vi "Format&SaveDataCleanbckp.vi"(0 "Data_Angle_deg":sgl[](array[numeric])=[490.08, 490.12, 490.16, 490.2], 1 "Measurement type":T4(ring)=enum."Contrast", 2 "Spectrum Custom Mode":u16(ring)=1 caption="Detector" items=["PD 1", "APD 1", "APD 2", "APD 1+2", "PD 2"], 3 "Suppl_2D":dbl[][](array[numeric]), 4 "Params Save":T3, 5 "DotNum":dbl, 6 "Data_PLInt_cts":i32[](array[numeric])=[1, 3, 2, 1], 7 "Main 3D Data to write":dbl[][][](array[numeric])=[[[2.2, 4.4, 3.3, 5.5, 6.6]]], 10 "Params XY Map SubVI":T1, 11 "Suppl":dbl[](array[numeric]), 12 "Data_FSMPos_V":dbl[][](array[numeric]), 14 "Data_CCD_px":dbl[][](array[numeric]), 15 "L2Exc_deg":dbl[](array[numeric]), 17 "L2Det_deg":dbl[](array[numeric]), 19 "Suppl_3D":dbl[][][](array[numeric])) -> (9 "datasetnumber":string, 13 "Log File Out":string, 16 "FullComment":string, 18 "WrittenDatasetName":string)   [LabVIEW 2019]
uses:
  TypeDefs/AcqMode.ctl
  <vilib>/UPVI/lvhdf5/dataset.llb/LVH5D Operation.ctl
  <vilib>/Utility/miscctls.llb/LVRectTypeDef.ctl
  <vilib>/UPVI/lvhdf5/attribute.llb/LVH5A Operation.ctl
  <vilib>/UPVI/lvhdf5/group.llb/H5G_obj_t.ctl
  <vilib>/UPVI/lvhdf5/identifier.llb/Not an HDF5 Refnum Constant.vi
  <vilib>/UPVI/lvhdf5/common.llb/To HDF5 Ref.vi
  <vilib>/UPVI/lvhdf5/group.llb/OpenCreateGroup (String).vi
  <vilib>/Utility/VariantDataType/GetClusterInfo.vi
  <vilib>/Utility/VariantDataType/GetTypeInfo.vi
  <vilib>/UPVI/lvhdf5/utility.llb/Select HDF5 Dialog.vi
  <vilib>/UPVI/lvhdf5/utility.llb/Select HDF5 Dialog (Object Only).vi
  <vilib>/UPVI/lvhdf5/dataset.llb/Simple H5Dwrite (Variant).vi
  <vilib>/UPVI/lvhdf5/attribute.llb/Write Multiple Attributes.vi
  <vilib>/UPVI/lvhdf5/dataset.llb/H5Dclose.vi
  <vilib>/UPVI/lvhdf5/dataset.llb/Write Dataset with Attributes.xnode
  <vilib>/UPVI/lvhdf5/library.llb/HDF5 Ref.ctl
  <vilib>/UPVI/lvhdf5/attribute.llb/Cluster to Attribute Array.xnode
  <vilib>/Utility/error.llb/Error Cluster From Error Code.vi
  <vilib>/UPVI/lvhdf5/dataset.llb/OpenCreateReplace Dataset by Element Type.vi
  <vilib>/UPVI/lvhdf5/dataspace.llb/H5Sselect_hyperslab.vi
  <vilib>/UPVI/lvhdf5/dataset.llb/H5Dwrite (Variant).vi
  <vilib>/UPVI/lvhdf5/dataset.llb/H5Dget_space.vi
  <vilib>/UPVI/lvhdf5/attribute.llb/private/LVH5AwriteWDTAttrs.vi
  <vilib>/UPVI/lvhdf5/dataspace.llb/H5Sclose.vi
  <vilib>/UPVI/lvhdf5/file.llb/LVH5F Operation.ctl
  <vilib>/UPVI/lvhdf5/utility.llb/Select HDF5 Dialog (File and Object).vi
  <vilib>/Utility/VariantDataType/VariantType.lvlib
panel:
  out "resulting string":string
  out "XyMap Params 2":dbl[][](array[numeric])
  out "SamplePrep":string
  out "SynthSolv":string
  out "SynthPolymPerc":dbl
  out "SynthPolym":string
  out "SynthDilution":dbl
  out "SynthTemp":dbl
  out "SynthName":string
  out "SampleOf":string
  out "SamplePrepdate":timestamp
  out "Detector":string
  out "Marker":i8[](array[numeric])
  out "FSM":dbl[](array[numeric])
  out "Att":dbl[](array[numeric])
  out "AttY":dbl
  out "AttX":dbl
  out "AttZ":dbl
  out "MarkerY":i8
  out "MarkerX":i8
  out "FSMx":dbl
  out "FSMy":dbl
  out "Grating":string
  in  "ESource":enum16{"P", "CW", "SK"}(ring)
  in  "Acq Mode":T2=enum."Spectrum" caption="Acq mode"
  in  "Log File In":string
  out "File path":path=path "Cluster Attributes.hdf5"
  in  "DatasetName":string="test"
  in  "Main 2D Data to write":dbl[][](array[numeric])=[[2.2, 4.4, 3.3, 5.5, 6.6]]
  in  "Comment":string="This is a test"
  out "Date":string="2006-1-11"
  in  "T_K":dbl=5.0
  in  "EPow_uW":dbl=0.21
  in  "EWL_nm":dbl=450.0
  in  "Time_ms":dbl=500.0
  in  "Det_Mono1_EntSlit_mm":dbl=0.01
  in  "Det_Mono1_ExtSlit_mm":dbl=0.01
  in  "WL_nm":sgl[](array[numeric])=[490.08, 490.12, 490.16, 490.2]
  in  "MeasurementName":string
  in  "FileName":string="test"
  in  "Det_Mono1_CenterWL_nm":dbl=490.0
  out "Exists":bool
  out "Homonyms":string[](array[string])
  out "size(s)":i32
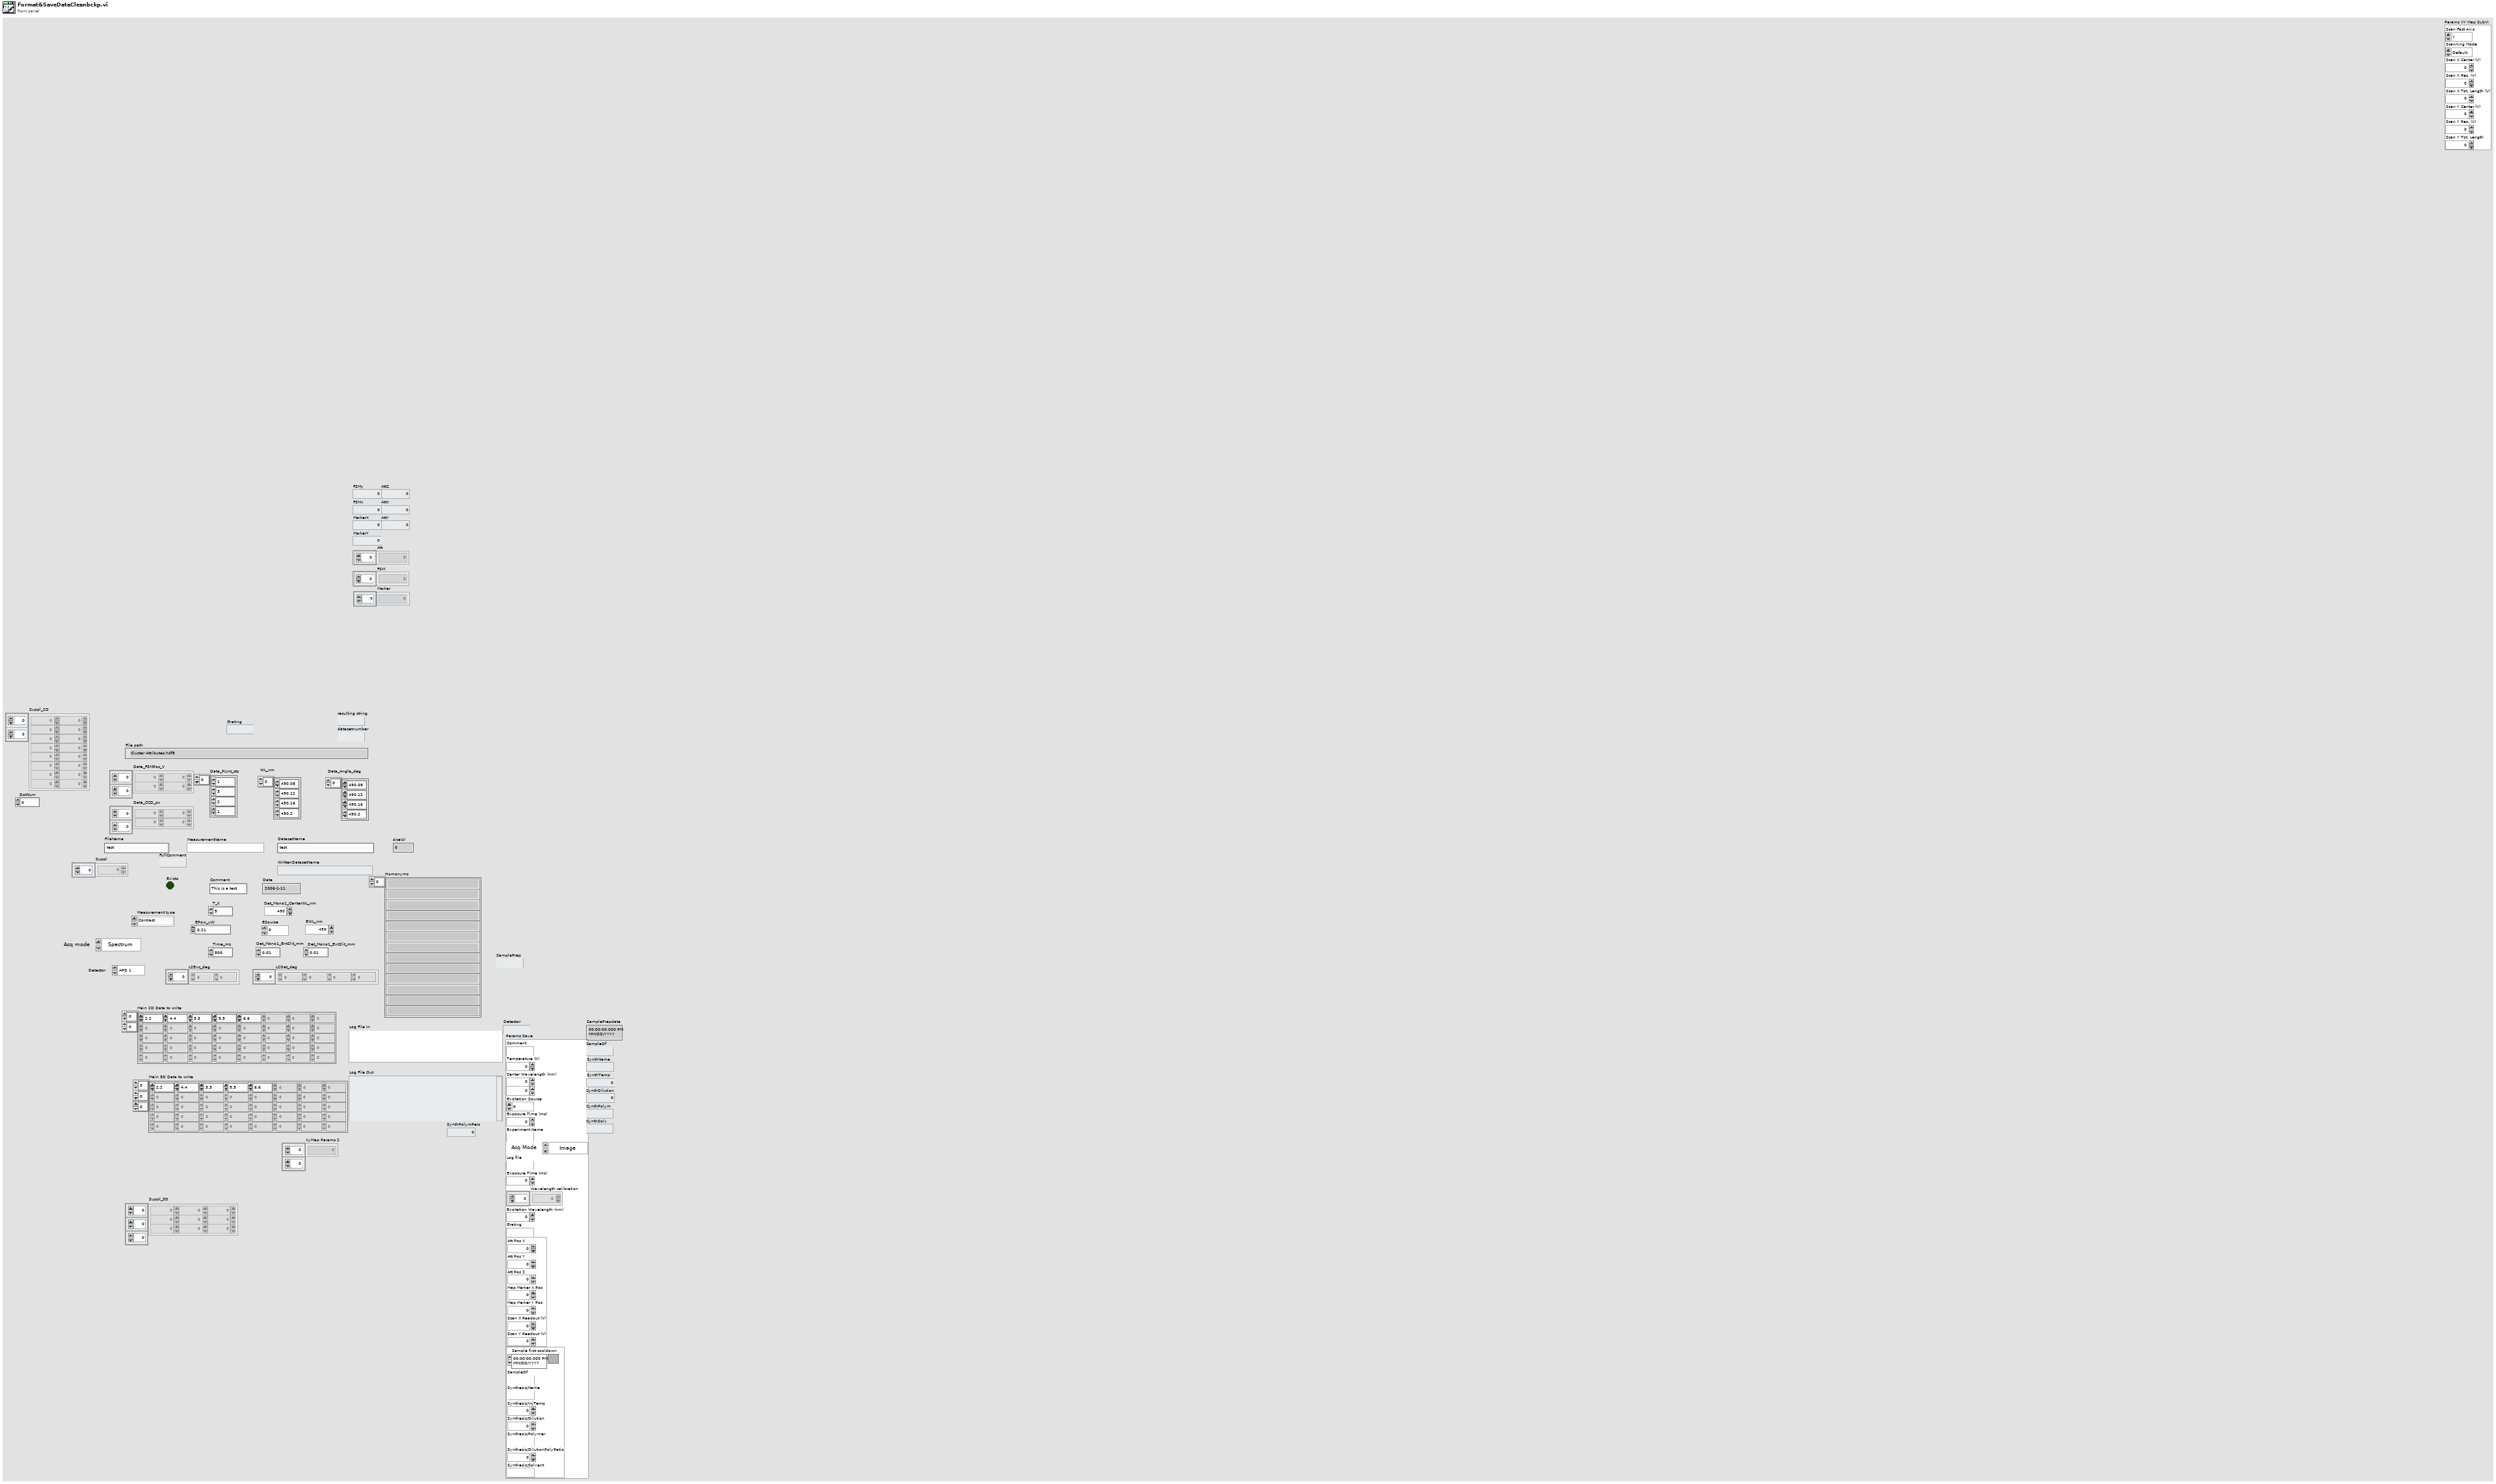
[diagram p1: front panel]
types:
  T1 = cluster{"Scan Fast Axis":enum16{"Y", "X"}, "Scanning Mode":enum16{"Default", "Snail", "Random", "Snake", "Line"}, "Scan X Center (V)":dbl, "Scan X Res. (V)":dbl, "Scan X Tot. Length (V)":dbl, "Scan Y Center (V)":dbl, "Scan Y Res. (V)":dbl, "Scan Y Tot. Length":dbl}
  T2 = typedef "AcqMode.ctl" = enum16{"Image", "Spectrum", "APD 1", "APD 2", "APD 1+2"}
  T3 = cluster{"Comment":string, "Temperature (K)":dbl, "Center Wavelength (nm)":dbl, "Numeric":dbl, "Excitation Source":enum16{"P", "CW", "SK"}, "Exposure Time (ms)":dbl, "Experiment Name":string, "Acq Mode":T2, "Log file":string, "Exposure Time (ms)":dbl, "Wavelength calibration":dbl[], "Excitation Wavelength (nm)":dbl, "Grating":string, "Cluster":cluster{"Att Pos X":dbl, "Att Pos Y":dbl, "Att Pos Z":dbl, "Map Marker X Pos":i8, "Map Marker Y Pos":i8, "Scan X Readout (V)":dbl, "Scan Y Readout (V)":dbl}, "Cluster":cluster{"Sample first cooldown":timestamp, "SampleOf":string, "Synthesis/Name":string, "Synthesis/InjTemp":dbl, "Synthesis/Dilution":dbl, "Synthesis/Polymer":string, "Synthesis/DilutionPolyRatio":dbl, "Synthesis/Solvent":string}}
  T4 = enum16{"Time Trace", "Contrast", "XY Intensity Map", "Polarisation", "Spectrum", "Michelson", "fPow", "PLE"}
  T5 = typedef "LVH5D Operation.ctl" = enum16{"open", "replace", "create", "open or create", "create or replace", "create or replace with confirmation"}
  T6 = typedef "LVH5A Operation.ctl" = enum16{"open", "replace", "create", "open or create", "create or replace", "create or replace with confirmation"}
  T7 = typedef "LVRectTypeDef.ctl" = cluster{"Left":i16, "Top":i16, "Right":i16, "Bottom":i16}
  T8 = cluster{"Behavior":enum32{"Invalid", "Default", "Floating", "Floating/Auto-Hide", "Modal"}, "Position":T7, "Center":bool, "Title":string}
  T9 = typedef "LVH5F Operation.ctl" = enum16{"open", "open or create", "create or replace", "create or replace (with confirmation)", "create", "open (read only)"}
  T10 = typedef "H5G_obj_t.ctl" = i32
  T11 = cluster{"Object Types (any)":T10[], "Object Pattern":string}
  T12 = cluster{"Att Pos X":dbl, "Att Pos Y":dbl, "Att Pos Z":dbl, "Map Marker X Pos":i8, "Map Marker Y Pos":i8, "Scan X Readout (V)":dbl, "Scan Y Readout (V)":dbl}
  T13 = cluster{"Sample first cooldown":timestamp, "SampleOf":string, "Synthesis/Name":string, "Synthesis/InjTemp":dbl, "Synthesis/Dilution":dbl, "Synthesis/Polymer":string, "Synthesis/DilutionPolyRatio":dbl, "Synthesis/Solvent":string}
  T14 = typedef "HDF5 Ref.ctl" = refnum<k1>
  T15 = cluster{"Date":string, "Comment":string, "T_K":dbl, "ESource":enum16{"P", "CW", "SK"}, "EWL_nm":dbl, "EPow_uW":dbl, "Time_ms":dbl, "WL_nm":sgl[], "Suppl":dbl[], "L2Exc_deg":dbl[], "L2Det_deg":dbl[], "Att":dbl[], "FSM":dbl[], "Marker":i8[], "Detector":string, "Grating":string, "SamplePrep":string, "SampleOf":string, "SynthName":string, "SynthTemp":dbl, "SynthDilution":dbl, "SynthPolym":string, "SynthPolymPerc":dbl, "SynthSolv":string}
  T16 = cluster{"Date":string, "Comment":string, "T_K":dbl, "ESource":enum16{"P", "CW", "SK"}, "EWL_nm":dbl, "EPow_uW":dbl, "Time_ms":dbl, "WL_nm":sgl[], "Suppl":dbl[], "L2Exc_deg":dbl[], "L2Det_deg":dbl[], "Suppl_2D":dbl[], "Att":dbl[], "FSM":dbl[], "Marker":i8[], "Detector":string, "Grating":string, "SamplePrep":string, "SampleOf":string, "SynthName":string, "SynthTemp":dbl, "SynthDilution":dbl, "SynthPolym":string, "SynthPolymPerc":dbl, "SynthSolv":string}
  T17 = cluster{"Date":string, "Comment":string, "T_K":dbl, "ESource":enum16{"P", "CW", "SK"}, "EWL_nm":dbl, "EPow_uW":dbl, "Time_ms":dbl, "WL_nm":sgl[], "Suppl":dbl[], "L2Exc_deg":dbl[], "L2Det_deg":dbl[], "Suppl_2D":dbl[][], "Att":dbl[], "FSM":dbl[], "Marker":i8[], "Detector":string, "Grating":string, "SamplePrep":string, "SampleOf":string, "SynthName":string, "SynthTemp":dbl, "SynthDilution":dbl, "SynthPolym":string, "SynthPolymPerc":dbl, "SynthSolv":string}
  T18 = cluster{"Date":string, "Comment":string, "T_K":dbl, "ESource":enum16{"P", "CW", "SK"}, "EWL_nm":dbl, "EPow_uW":dbl, "Time_ms":dbl, "WL_nm":sgl[], "Suppl_2D":dbl[][], "L2Exc_deg":dbl[], "L2Det_deg":dbl[], "Att":dbl[], "FSM":dbl[], "Marker":i8[], "Detector":string, "Grating":string, "SamplePrep":string, "SampleOf":string, "SynthName":string, "SynthTemp":dbl, "SynthDilution":dbl, "SynthPolym":string, "SynthPolymPerc":dbl, "SynthSolv":string}
  T19 = cluster{"Date":string, "Comment":string, "T_K":dbl, "ESource":enum16{"P", "CW", "SK"}, "EWL_nm":dbl, "EPow_uW":dbl, "Time_ms":dbl, "WL_nm":sgl[], "Suppl_3D":dbl[][][], "L2Exc_deg":dbl[], "L2Det_deg":dbl[], "Att":dbl[], "FSM":dbl[], "Marker":i8[], "Detector":string, "Grating":string, "SamplePrep":string, "SampleOf":string, "SynthName":string, "SynthTemp":dbl, "SynthDilution":dbl, "SynthPolym":string, "SynthPolymPerc":dbl, "SynthSolv":string}
  T20 = cluster{"Date":string, "Comment":string, "T_K":dbl, "ESource":enum16{"P", "CW", "SK"}, "EWL_nm":dbl, "EPow_uW":dbl, "Time_ms":dbl, "WL_nm":sgl[], "Suppl":dbl[], "L2Exc_deg":dbl[], "L2Det_deg":dbl[], "Att":dbl[], "FSM":dbl[], "Marker":i8[], "SamplePrep":string, "SampleOf":string, "SynthName":string, "SynthTemp":dbl, "SynthDilution":dbl, "SynthPolym":string, "SynthPolymPerc":dbl, "SynthSolv":string}
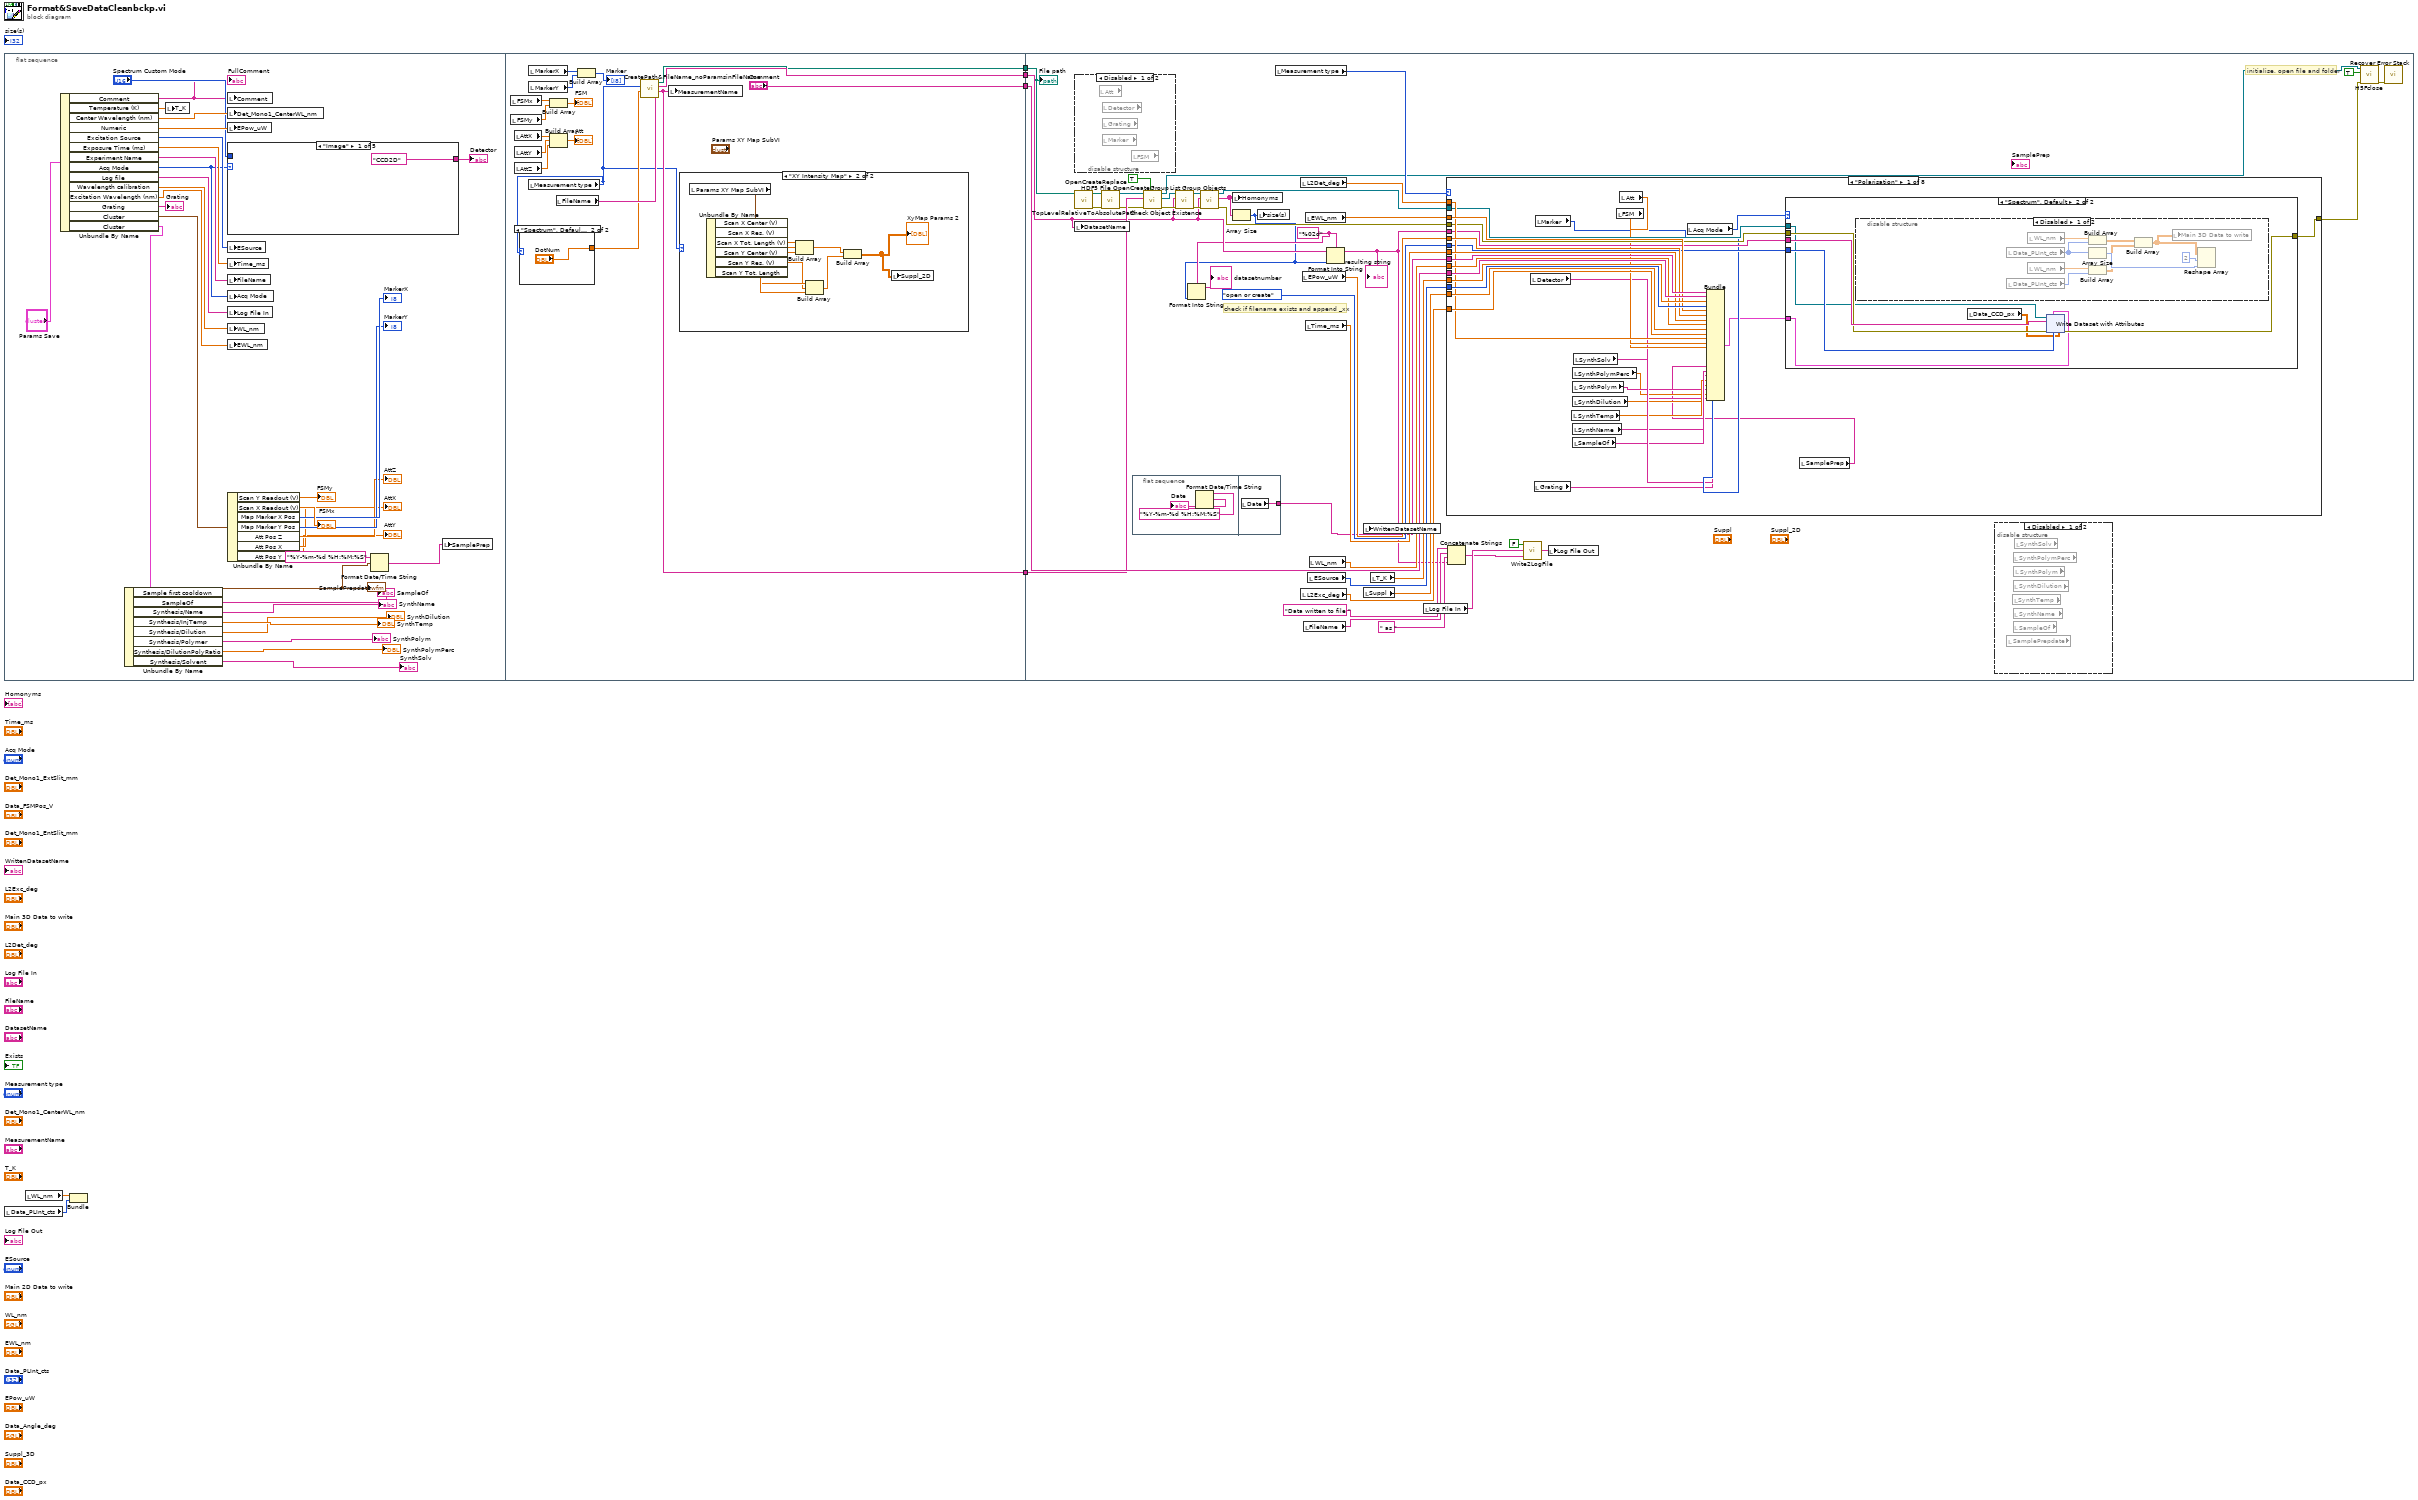
[diagram p0: block diagram]
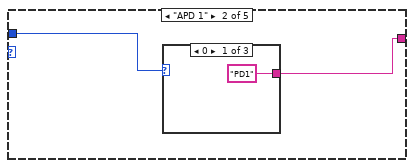
[diagram p2: hidden frame]
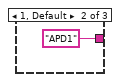
[diagram p3: hidden frame]
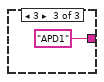
[diagram p4: hidden frame]
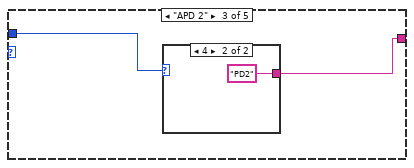
[diagram p5: hidden frame]
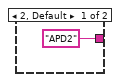
[diagram p6: hidden frame]
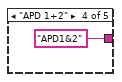
[diagram p7: hidden frame]
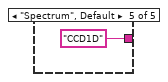
[diagram p8: hidden frame]
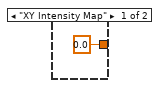
[diagram p9: hidden frame]
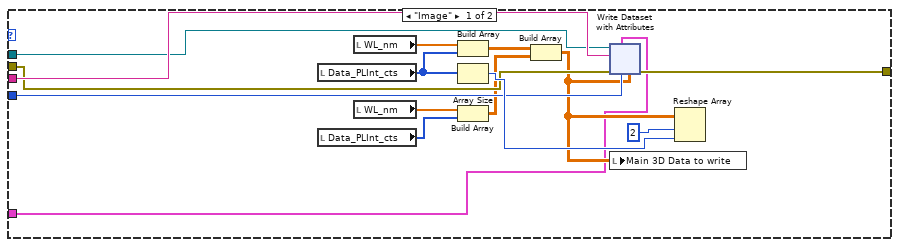
[diagram p13: hidden frame]
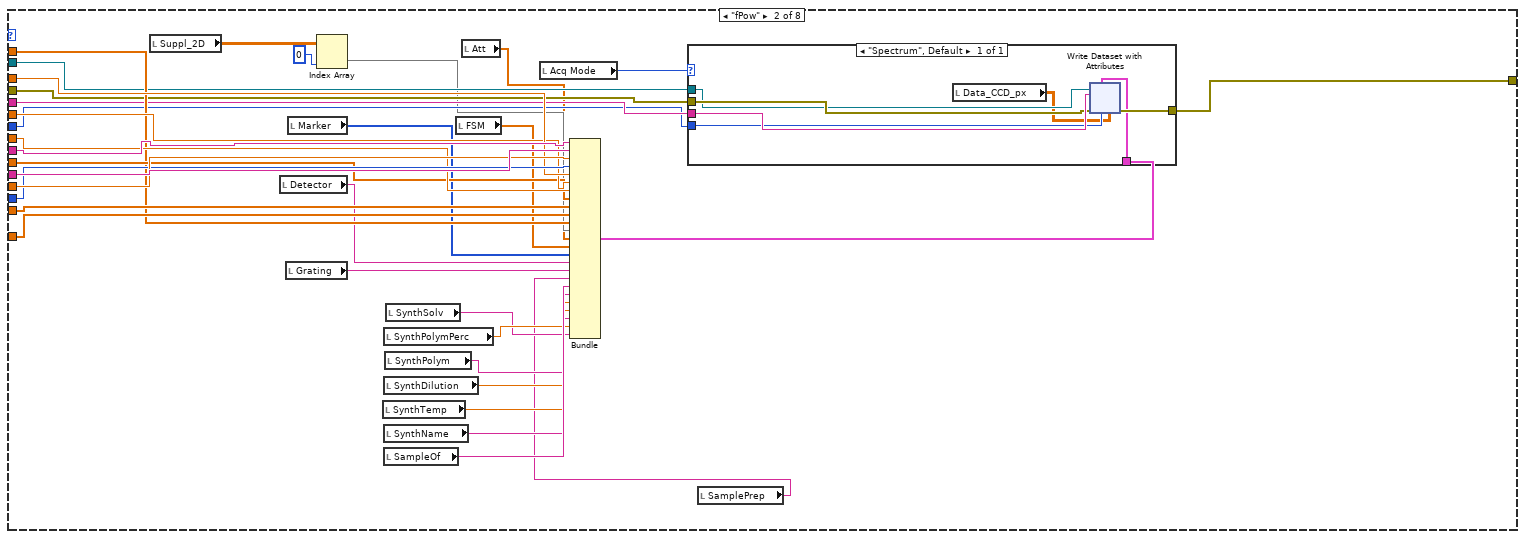
[diagram p15: hidden frame]
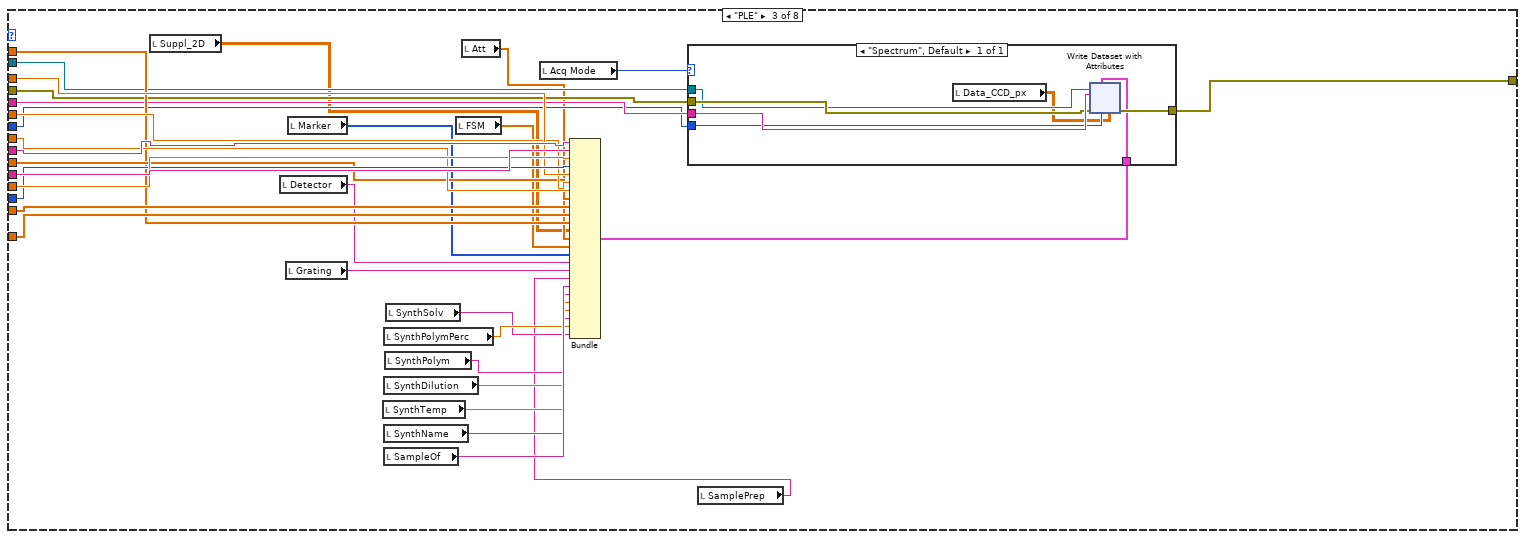
[diagram p16: hidden frame]
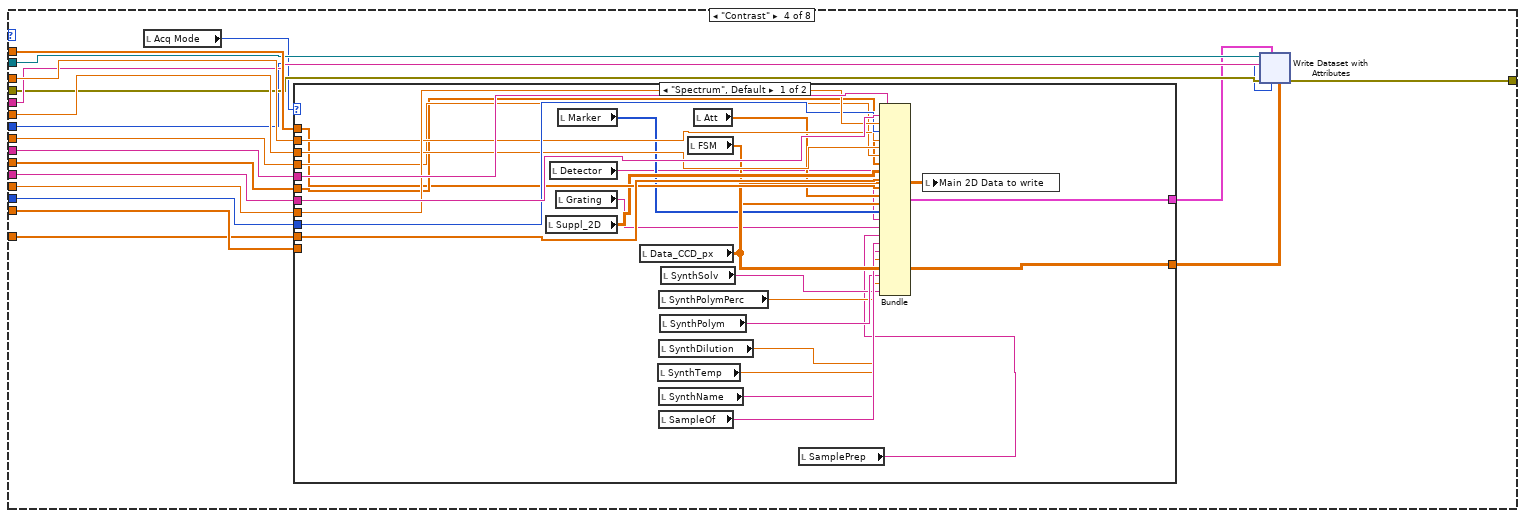
[diagram p17: hidden frame]
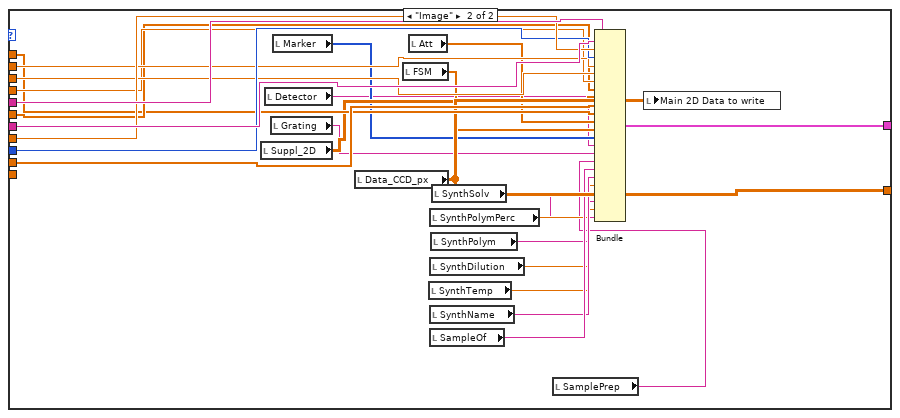
[diagram p18: hidden frame]
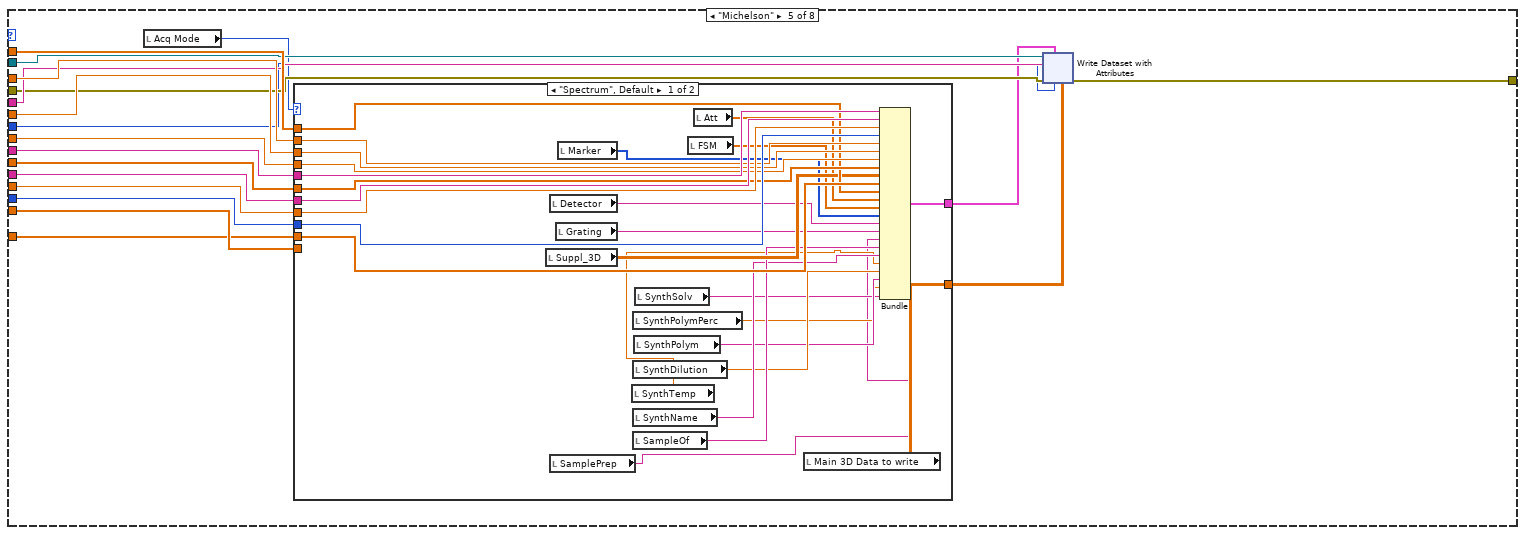
[diagram p19: hidden frame]
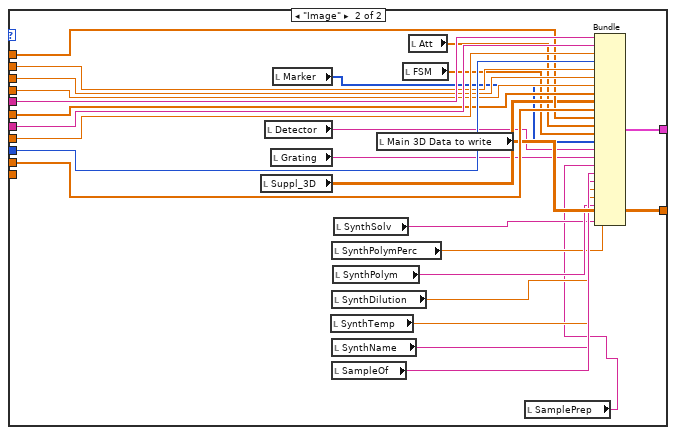
[diagram p20: hidden frame]
diagram:
  n1 = flat-sequence {
    tunnel: ["Comment"] -> w4
    tunnel: [w68] -> w3
    tunnel: [w67] -> w2
    tunnel: [w66] -> w1
    tunnel: w4 -> [w111]
    tunnel: w3 -> [w87]
    tunnel: w2 -> [w103]
    tunnel: w1 -> [w82]
    frame #0 {
      n2 = Unbundle By Name("Params Save") -> ("Comment"=w19:string, "Temperature (K)"=w40:dbl, "Center Wavelength (nm)"=w38:dbl, "Numeric"=w39:dbl, "Excitation Source"=w37:enum16{"P", "CW", "SK"}, "Exposure Time (ms)"=w36:dbl, "Experiment Name"=w34:string, "Acq Mode"=w31:T2, "Log file"=w35:string, "Wavelength calibration"=w32:dbl[], "Excitation Wavelength (nm)"=w33:dbl, "Grating"=→"Grating":string, "Cluster"=w27:T12, "Cluster"=w17:T13)
      "FullComment" <- w19
      n3 = Unbundle By Name(w17) -> ("Sample first cooldown"=w8:timestamp, "SampleOf"=→"SampleOf":string, "Synthesis/Name"=→"SynthName":string, "Synthesis/InjTemp"=→"SynthTemp":dbl, "Synthesis/Dilution"=→"SynthDilution":dbl, "Synthesis/Polymer"=→"SynthPolym":string, "Synthesis/DilutionPolyRatio"=→"SynthPolymPerc":dbl, "Synthesis/Solvent"=→"SynthSolv":string)
      "SamplePrepdate" <- w8
      n4 = local write "T_K"(w40) -> ()
      n5 = local write "Comment"(w19) -> ()
      n6 = local write "Det_Mono1_CenterWL_nm"(w38) -> ()
      n7 = local write "EPow_uW"(w39) -> ()
      n8 = case shown="\"Image\"" w31 {
        tunnel: ["CCD2D" w43 w48 "APD1&2" "CCD1D"] -> w29
        tunnel: "Spectrum Custom Mode" -> [_ w42 w47 _ _]
        frame "Image" {
        }
        frame "APD 1" {
          n9 = case shown="0" w42 {
            tunnel: ["PD1" "APD1" "APD1"] -> w43
            frame 0 {
            }
            frame 1, Default {
            }
            frame 3 {
            }
          }
        }
        frame "APD 2" {
          n10 = case shown="4" w47 {
            tunnel: ["APD2" "PD2"] -> w48
            frame 2, Default {
            }
            frame 4 {
            }
          }
        }
        frame "APD 1+2" {
        }
        frame "Spectrum", Default {
        }
      }
      "Detector" <- w29
      n11 = local write "ESource"(w37) -> ()
      n12 = local write "Time_ms"(w36) -> ()
      n13 = local write "FileName"(w34) -> ()
      n14 = local write "Acq Mode"(w31) -> ()
      n15 = local write "Log File In"(w35) -> ()
      n16 = local write "WL_nm"(w32) -> ()
      n17 = local write "EWL_nm"(w33) -> ()
      n18 = Unbundle By Name(w27) -> ("Scan Y Readout (V)"=→"FSMy":dbl, "Scan X Readout (V)"=→"FSMx":dbl, "Map Marker X Pos"=→"MarkerX":i8, "Map Marker Y Pos"=→"MarkerY":i8, "Att Pos Z"=→"AttZ":dbl, "Att Pos X"=→"AttX":dbl, "Att Pos Y"=→"AttY":dbl)
      n19 = Format Date/Time String(time format string (%c)="%Y-%m-%d %H:%M:%S", seconds (now)=w8) -> (date/time string=w7:string)  [unwired: 1 in]
      n20 = local write "SamplePrep"(w7) -> ()
    }
    frame #1 {
      n21 = local read "FSMx"() -> (w57:dbl)
      n22 = local read "FSMy"() -> (w58:dbl)
      n23 = local read "AttX"() -> (w54:dbl)
      n24 = local read "AttY"() -> (w55:dbl)
      n25 = local read "AttZ"() -> (w56:dbl)
      n26 = local read "Measurement type"() -> (w53:T4)
      n27 = case shown="\"Spectrum\", Default" w53 {
        tunnel: [0.0 ("DotNum") "DotNum"] -> w64
        frame "XY Intensity Map" {
        }
        frame "Spectrum", Default {
        }
      }
      n28 = local read "MarkerX"() -> (w59:i8)
      n29 = local read "MarkerY"() -> (w60:i8)
      n30 = Build Array(w57, w58) -> (→"FSM":dbl[])
      n31 = Build Array(w54, w55, w56) -> (→"Att":dbl[])
      n32 = local read "FileName"() -> (w65:string)
      n33 = Build Array(w59, w60) -> (→"Marker":i8[])
      n34 = call "CreatePath&FileName_noParamsinFileName.vi"("FileName"=w65, "DotNum"=w64, "Measurement type"=w53) -> ("MeasurementGroupName"=w67:string, "DatasetName"=w68:string, "File path"=w66:path)  [unwired: 3 in]
      n35 = local write "MeasurementName"(w67) -> ()
      n36 = case shown="\"XY Intensity Map\"" w53 {
        frame "Polarisation", Default {
        }
        frame "XY Intensity Map" {
          n37 = local read "Params XY Map SubVI"() -> (w81:T1)
          n38 = Unbundle By Name(w81) -> ("Scan X Center (V)"=w80:dbl, "Scan X Res. (V)"=w79:dbl, "Scan X Tot. Length (V)"=w78:dbl, "Scan Y Center (V)"=w76:dbl, "Scan Y Res. (V)"=w75:dbl, "Scan Y Tot. Length"=w77:dbl)
          n39 = Build Array(w80, w79, w78) -> (w74:dbl[])
          n40 = Build Array(w76, w75, w77) -> (w73:dbl[])
          n41 = Build Array(w74, w73) -> (w72:dbl[][])
          "XyMap Params 2" <- w72
          n42 = local write "Suppl_2D"(w72) -> ()
        }
      }
    }
    frame #2 {
      w85 = "%02d" ("format string")
      # "initialise, open file and folder"
      # "check if filename exists and append _xx"
      n43 = disable-structure shown="Disabled" {
        frame Disabled {
          n44 = local read "Att"() -> ()  [unwired: 1 out]
          n45 = local read "Detector"() -> ()  [unwired: 1 out]
          n46 = local read "Grating"() -> ()  [unwired: 1 out]
          n47 = local read "Marker"() -> ()  [unwired: 1 out]
          n48 = local read "FSM"() -> ()  [unwired: 1 out]
        }
        frame Enabled {
        }
      }
      n49 = call "TopLevelRelativeToAbsolutePath.vi"("Path Relative to Top Level VI"=w82) -> ("error out"=w96:errorcluster, "Absolute path"=w95:path)  [unwired: 9 in]
      n50 = local write "DatasetName"(w87) -> ()
      n51 = call <vilib>:"OpenCreateReplace HDF5 File.vi"("error in (no error)"=w96, "path"=w95) -> ("error out"=w98:errorcluster, "HDF5 Ref out"=w97:T14)  [unwired: 6 in]
      n52 = flat-sequence {
        tunnel: [w127] -> w110
        frame #0 {
          n53 = Format Date/Time String(time format string (%c)="%Y-%m-%d %H:%M:%S") -> (date/time string=→"Date":string)  [unwired: 2 in]
        }
        frame #1 {
          n54 = local read "Date"() -> (w127:string)
        }
      }
      n55 = call-poly <vilib>:"OpenCreateGroup.vi"("Create if not found (F)"=TRUE, "error in (no error)"=w98, "Group"=w103, "HDF5 Ref"=w97) -> ("error out"=w106:errorcluster, "HDF5 Group Ref"=w105:T14, "HDF5 Ref out"=w101:T14)  [unwired: 5 in]
      n56 = call <vilib>:"Check Object Existence.vi"("error in (no error)"=w106, "name"=w87, "HDF5 Ref"=w105) -> ("error out"=w107:errorcluster, "HDF5 Ref out"=w108:T14)  [unwired: 4 in, 1 out]
      n57 = call <vilib>:"List Group Objects.vi"("error in (no error)"=w107, "pattern"=w87, "HDF5 Loc Ref"=w108) -> ("error out"=w121:errorcluster, "Object Names"=w109:string[], "HDF5 Loc Ref out"=w123:T14)  [unwired: 3 in, 1 out]
      n58 = local write "Homonyms"(w109) -> ()
      n59 = Array Size(array=w109) -> (size(s)=w84:i32)
      n60 = Format Into String(format string=w85, w84) -> (resulting string=→"datasetnumber":string)  [unwired: 2 in, 1 out]
      n61 = local write "size(s)"(w84) -> ()
      n62 = local read "Measurement type"() -> (w102:T4)
      n63 = local read "L2Det_deg"() -> (w120:dbl[])
      n64 = local read "L2Exc_deg"() -> (w119:dbl[])
      n65 = local read "EPow_uW"() -> (w115:dbl)
      n66 = local read "FileName"() -> (w93:string)
      n67 = local read "EWL_nm"() -> (w114:dbl)
      n68 = local read "Time_ms"() -> (w116:dbl)
      n69 = local read "ESource"() -> (w113:enum16{"P", "CW", "SK"})
      n70 = local read "WL_nm"() -> (w117:sgl[])
      n71 = Format Into String(format string=w85, initial string=w87, w84) -> (resulting string=w91:string)  [unwired: 1 in, 1 out]
      "resulting string" <- w91
      n72 = local write "WrittenDatasetName"(w91) -> ()
      n73 = local read "Suppl"() -> (w118:dbl[])
      n74 = local read "T_K"() -> (w112:dbl)
      n75 = local read "Log File In"() -> (w90:string)
      n76 = case shown="\"Polarisation\"" w102 {
        tunnel: w110 -> [w158 w903 w1284 w1652 w2063 w2472 w4298 w5066]
        tunnel: w111 -> [w157 w902 w1283 w1651 w2062 w2471 w4297 w5065]
        tunnel: w112 -> [w156 w901 w1282 w1650 w2061 w2470 w4296 w5064]
        tunnel: w113 -> [w155 w900 w1281 w1649 w2060 w2469 w4295 w5063]
        tunnel: w114 -> [w154 w899 w1280 w1648 w2059 w2468 w4294 w5062]
        tunnel: w115 -> [w153 w898 w1279 w1647 w2058 w2467 w4293 w5061]
        tunnel: w116 -> [w152 w897 w1278 w1646 w2057 w2466 w4292 w5060]
        tunnel: w117 -> [w151 w896 w1277 w1645 w2056 w2465 w4291 w5059]
        tunnel: w118 -> [w150 w895 w1276 w1644 w2055 w2464 w4290 w5058]
        tunnel: w119 -> [w149 w894 w1275 w1643 w2054 w2463 w4289 w5057]
        tunnel: w120 -> [w148 w893 w1274 w1642 w2053 w2462 w4288 w5056]
        tunnel: w91 -> [w147 w892 w1273 w1641 w2052 w2461 w4287 w5055]
        tunnel: w121 -> [w146 w891 w1272 w1640 w2051 w2460 w4286 w5054]
        tunnel: LVH5D_Operation."open or create" ("operation (open or create)") -> [w145 w890 w1271 w1639 w2050 w2459 w4285 w5053]
        tunnel: w123 -> [w144 w889 w1270 w1638 w2049 w2458 w4284 w5052]
        tunnel: [w143 w888 w1269 w1637 w2048 w2457 w4283 w5051] -> w124
        frame "Polarisation" {
          n77 = local read "Detector"() -> (w138:string)
          n78 = local read "Grating"() -> (w137:string)
          n79 = local read "Marker"() -> (w139:i8[])
          n80 = local read "SynthTemp"() -> (w134:dbl)
          n81 = local read "SynthPolymPerc"() -> (w131:dbl)
          n82 = local read "SynthDilution"() -> (w133:dbl)
          n83 = local read "SynthName"() -> (w135:string)
          n84 = local read "SampleOf"() -> (w136:string)
          n85 = local read "SynthPolym"() -> (w132:string)
          n86 = local read "SynthSolv"() -> (w130:string)
          n87 = local read "FSM"() -> (w140:dbl[])
          n88 = local read "Att"() -> (w141:dbl[])
          n89 = local read "Acq Mode"() -> (w142:T2)
          n90 = local read "SamplePrep"() -> (w128:string)
          n91 = Bundle("Date"=w158, "Comment"=w157, "T_K"=w156, "ESource"=w155, "EWL_nm"=w154, "EPow_uW"=w153, "Time_ms"=w152, "WL_nm"=w151, "Suppl"=w150, "L2Exc_deg"=w149, "L2Det_deg"=w148, "Att"=w141, "FSM"=w140, "Marker"=w139, "Detector"=w138, "Grating"=w137, "SamplePrep"=w128, "SampleOf"=w136, "SynthName"=w135, "SynthTemp"=w134, "SynthDilution"=w133, "SynthPolym"=w132, "SynthPolymPerc"=w131, "SynthSolv"=w130) -> (w129:T15)  [unwired: 1 in]
          n92 = case shown="\"Spectrum\", Default" w142 {
            tunnel: w147 -> [w169 w520]
            tunnel: w146 -> [w168 w519]
            tunnel: w145 -> [w167 w518]
            tunnel: w144 -> [w166 w517]
            tunnel: [w165 w516] -> w143
            tunnel: w129 -> [w159 w514]
            frame "Image" {
              n93 = local read "Data_PLInt_cts"() -> (w171:i32[])
              n94 = local read "Data_PLInt_cts"() -> (w163:i32[])
              n95 = local read "WL_nm"() -> (w170:sgl[])
              n96 = local read "WL_nm"() -> (w164:sgl[])
              n97 = Build Array(w170, w171) -> (w161:sgl[][])
              n98 = Array Size(array=w171) -> (size(s)=w172:i32)
              n99 = Build Array(w164, w163) -> (w162:sgl[][])
              n100 = Build Array(w161, w162) -> (w160:sgl[][][])
              n101 = xnode "Write Dataset with Attributes"("Dataset Path"=w169, "error in (no error)"=w168, "operation (open or create)"=w167, "HDF5 Path or Ref"=w166, "Attribute Value(s)"=w159, "Data"=w160) -> ("error out"=w165:errorcluster)  [unwired: 2 in, 2 out]
              n102 = local write "Main 3D Data to write"(w160) -> ()
              n103 = Reshape Array(w160, 2 ("dimension size"), w172) -> ()  [unwired: 1 out]
            }
            frame "Spectrum", Default {
              n104 = disable-structure shown="Disabled" {
                frame Disabled {
                  n105 = local read "Data_PLInt_cts"() -> (w527:i32[])
                  n106 = local read "Data_PLInt_cts"() -> (w524:i32[])
                  n107 = local read "WL_nm"() -> (w526:sgl[])
                  n108 = local read "WL_nm"() -> (w525:sgl[])
                  n109 = Build Array(w526, w527) -> (w522:sgl[][])
                  n110 = Array Size(array=w527) -> (size(s)=w528:i32)
                  n111 = Build Array(w525, w524) -> (w523:sgl[][])
                  n112 = Build Array(w522, w523) -> (w521:sgl[][][])
                  n113 = local write "Main 3D Data to write"(w521) -> ()
                  n114 = Reshape Array(w521, 2 ("dimension size"), w528) -> ()  [unwired: 1 out]
                }
                frame Enabled {
                }
              }
              n115 = local read "Data_CCD_px"() -> (w515:dbl[][])
              n116 = xnode "Write Dataset with Attributes"("Dataset Path"=w520, "error in (no error)"=w519, "operation (open or create)"=w518, "HDF5 Path or Ref"=w517, "Attribute Value(s)"=w514, "Data"=w515) -> ("error out"=w516:errorcluster)  [unwired: 2 in, 2 out]
            }
          }
        }
        frame "fPow" {
          n117 = local read "Suppl_2D"() -> (w886:dbl[][])
          n118 = local read "Detector"() -> (w880:string)
          n119 = local read "Grating"() -> (w879:string)
          n120 = local read "Marker"() -> (w881:i8[])
          n121 = Index Array(array=w886, index (col)=0 ("disabled index (col)")) -> (element=w884:dbl[])  [unwired: 1 in]
          n122 = local read "SynthTemp"() -> (w876:dbl)
          n123 = local read "SynthPolymPerc"() -> (w873:dbl)
          n124 = local read "SynthDilution"() -> (w875:dbl)
          n125 = local read "SynthName"() -> (w877:string)
          n126 = local read "SampleOf"() -> (w878:string)
          n127 = local read "SynthPolym"() -> (w874:string)
          n128 = local read "SynthSolv"() -> (w872:string)
          n129 = local read "FSM"() -> (w882:dbl[])
          n130 = local read "Att"() -> (w883:dbl[])
          n131 = local read "Acq Mode"() -> (w887:T2)
          n132 = local read "SamplePrep"() -> (w870:string)
          n133 = Bundle("Date"=w903, "Comment"=w902, "T_K"=w901, "ESource"=w900, "EWL_nm"=w899, "EPow_uW"=w898, "Time_ms"=w897, "WL_nm"=w896, "Suppl"=w895, "L2Exc_deg"=w894, "L2Det_deg"=w893, "Suppl_2D"=w884, "Att"=w883, "FSM"=w882, "Marker"=w881, "Detector"=w880, "Grating"=w879, "SamplePrep"=w870, "SampleOf"=w878, "SynthName"=w877, "SynthTemp"=w876, "SynthDilution"=w875, "SynthPolym"=w874, "SynthPolymPerc"=w873, "SynthSolv"=w872) -> (w871:T16)  [unwired: 1 in]
          n134 = case shown="\"Spectrum\", Default" w887 {
            tunnel: w892 -> [w910]
            tunnel: w891 -> [w909]
            tunnel: w890 -> [w908]
            tunnel: w889 -> [w907]
            tunnel: [w906] -> w888
            tunnel: w871 -> [w904]
            frame "Spectrum", Default {
              n135 = local read "Data_CCD_px"() -> (w905:dbl[][])
              n136 = xnode "Write Dataset with Attributes"("Dataset Path"=w910, "error in (no error)"=w909, "operation (open or create)"=w908, "HDF5 Path or Ref"=w907, "Attribute Value(s)"=w904, "Data"=w905) -> ("error out"=w906:errorcluster)  [unwired: 2 in, 2 out]
            }
          }
        }
        frame "PLE" {
          n137 = local read "Suppl_2D"() -> (w1254:dbl[][])
          n138 = local read "Detector"() -> (w1264:string)
          n139 = local read "Grating"() -> (w1263:string)
          n140 = local read "Marker"() -> (w1265:i8[])
          n141 = local read "SynthTemp"() -> (w1260:dbl)
          n142 = local read "SynthPolymPerc"() -> (w1257:dbl)
          n143 = local read "SynthDilution"() -> (w1259:dbl)
          n144 = local read "SynthName"() -> (w1261:string)
          n145 = local read "SampleOf"() -> (w1262:string)
          n146 = local read "SynthPolym"() -> (w1258:string)
          n147 = local read "SynthSolv"() -> (w1256:string)
          n148 = local read "FSM"() -> (w1266:dbl[])
          n149 = local read "Att"() -> (w1267:dbl[])
          n150 = local read "Acq Mode"() -> (w1268:T2)
          n151 = local read "SamplePrep"() -> (w1255:string)
          n152 = Bundle("Date"=w1284, "Comment"=w1283, "T_K"=w1282, "ESource"=w1281, "EWL_nm"=w1280, "EPow_uW"=w1279, "Time_ms"=w1278, "WL_nm"=w1277, "Suppl"=w1276, "L2Exc_deg"=w1275, "L2Det_deg"=w1274, "Suppl_2D"=w1254, "Att"=w1267, "FSM"=w1266, "Marker"=w1265, "Detector"=w1264, "Grating"=w1263, "SamplePrep"=w1255, "SampleOf"=w1262, "SynthName"=w1261, "SynthTemp"=w1260, "SynthDilution"=w1259, "SynthPolym"=w1258, "SynthPolymPerc"=w1257, "SynthSolv"=w1256) -> (w1253:T17)  [unwired: 1 in]
          n153 = case shown="\"Spectrum\", Default" w1268 {
            tunnel: w1273 -> [w1291]
            tunnel: w1272 -> [w1290]
            tunnel: w1271 -> [w1289]
            tunnel: w1270 -> [w1288]
            tunnel: [w1287] -> w1269
            tunnel: w1253 -> [w1285]
            frame "Spectrum", Default {
              n154 = local read "Data_CCD_px"() -> (w1286:dbl[][])
              n155 = xnode "Write Dataset with Attributes"("Dataset Path"=w1291, "error in (no error)"=w1290, "operation (open or create)"=w1289, "HDF5 Path or Ref"=w1288, "Attribute Value(s)"=w1285, "Data"=w1286) -> ("error out"=w1287:errorcluster)  [unwired: 2 in, 2 out]
            }
          }
        }
        frame "Contrast" {
          n156 = local read "Acq Mode"() -> (w1635:T2)
          n157 = case shown="\"Spectrum\", Default" w1635 {
            tunnel: w1652 -> [w1678 w1704]
            tunnel: w1651 -> [w1677 w1703]
            tunnel: w1650 -> [w1676 w1702]
            tunnel: w1649 -> [w1675 w1701]
            tunnel: w1648 -> [w1674 w1700]
            tunnel: w1647 -> [w1673 w1699]
            tunnel: w1646 -> [w1672 w1698]
            tunnel: w1645 -> [w1671 w1697]
            tunnel: w1644 -> [_ _]
            tunnel: w1643 -> [w1670 w1696]
            tunnel: w1642 -> [w1669 w1695]
            tunnel: [w1668 w1694] -> w1636
            tunnel: [w1654 w1680] -> w1634
            frame "Spectrum", Default {
              n158 = local read "Suppl_2D"() -> (w1667:dbl[][])
              n159 = local read "Detector"() -> (w1663:string)
              n160 = local read "Grating"() -> (w1662:string)
              n161 = local read "Marker"() -> (w1664:i8[])
              n162 = local read "Data_CCD_px"() -> (w1668:dbl[][])
              n163 = local read "SynthTemp"() -> (w1659:dbl)
              n164 = local read "SynthPolymPerc"() -> (w1656:dbl)
              n165 = local read "SynthDilution"() -> (w1658:dbl)
              n166 = local read "SynthName"() -> (w1660:string)
              n167 = local read "SampleOf"() -> (w1661:string)
              n168 = local read "SynthPolym"() -> (w1657:string)
              n169 = local read "SynthSolv"() -> (w1655:string)
              n170 = local read "FSM"() -> (w1665:dbl[])
              n171 = local read "Att"() -> (w1666:dbl[])
              n172 = local read "SamplePrep"() -> (w1653:string)
              n173 = Bundle("Date"=w1678, "Comment"=w1677, "T_K"=w1676, "ESource"=w1675, "EWL_nm"=w1674, "EPow_uW"=w1673, "Time_ms"=w1672, "WL_nm"=w1671, "Suppl_2D"=w1667, "L2Exc_deg"=w1670, "L2Det_deg"=w1669, "Att"=w1666, "FSM"=w1665, "Marker"=w1664, "Detector"=w1663, "Grating"=w1662, "SamplePrep"=w1653, "SampleOf"=w1661, "SynthName"=w1660, "SynthTemp"=w1659, "SynthDilution"=w1658, "SynthPolym"=w1657, "SynthPolymPerc"=w1656, "SynthSolv"=w1655) -> (w1654:T18)  [unwired: 1 in]
              n174 = local write "Main 2D Data to write"(w1668) -> ()
            }
            frame "Image" {
              n175 = local read "Suppl_2D"() -> (w1693:dbl[][])
              n176 = local read "Detector"() -> (w1689:string)
              n177 = local read "Grating"() -> (w1688:string)
              n178 = local read "Marker"() -> (w1690:i8[])
              n179 = local read "Data_CCD_px"() -> (w1694:dbl[][])
              n180 = local read "FSM"() -> (w1691:dbl[])
              n181 = local read "Att"() -> (w1692:dbl[])
              n182 = local read "SynthTemp"() -> (w1685:dbl)
              n183 = local read "SynthPolymPerc"() -> (w1682:dbl)
              n184 = local read "SynthDilution"() -> (w1684:dbl)
              n185 = local read "SynthName"() -> (w1686:string)
              n186 = local read "SampleOf"() -> (w1687:string)
              n187 = local read "SynthPolym"() -> (w1683:string)
              n188 = local read "SynthSolv"() -> (w1681:string)
              n189 = local read "SamplePrep"() -> (w1679:string)
              n190 = Bundle("Date"=w1704, "Comment"=w1703, "T_K"=w1702, "ESource"=w1701, "EWL_nm"=w1700, "EPow_uW"=w1699, "Time_ms"=w1698, "WL_nm"=w1697, "Suppl_2D"=w1693, "L2Exc_deg"=w1696, "L2Det_deg"=w1695, "Att"=w1692, "FSM"=w1691, "Marker"=w1690, "Detector"=w1689, "Grating"=w1688, "SamplePrep"=w1679, "SampleOf"=w1687, "SynthName"=w1686, "SynthTemp"=w1685, "SynthDilution"=w1684, "SynthPolym"=w1683, "SynthPolymPerc"=w1682, "SynthSolv"=w1681) -> (w1680:T18)  [unwired: 1 in]
              n191 = local write "Main 2D Data to write"(w1694) -> ()
            }
          }
          n192 = xnode "Write Dataset with Attributes"("Dataset Path"=w1641, "error in (no error)"=w1640, "operation (open or create)"=w1639, "HDF5 Path or Ref"=w1638, "Attribute Value(s)"=w1634, "Data"=w1636) -> ("error out"=w1637:errorcluster)  [unwired: 2 in, 2 out]
        }
        frame "Michelson" {
          n193 = local read "Acq Mode"() -> (w2046:T2)
          n194 = case shown="\"Spectrum\", Default" w2046 {
            tunnel: w2063 -> [w2089 w2115]
            tunnel: w2062 -> [w2088 w2114]
            tunnel: w2061 -> [w2087 w2113]
            tunnel: w2060 -> [w2086 w2112]
            tunnel: w2059 -> [w2085 w2111]
            tunnel: w2058 -> [w2084 w2110]
            tunnel: w2057 -> [w2083 w2109]
            tunnel: w2056 -> [w2082 w2108]
            tunnel: w2055 -> [_ _]
            tunnel: w2054 -> [w2081 w2107]
            tunnel: w2053 -> [w2080 w2106]
            tunnel: [w2079 w2105] -> w2047
            tunnel: [w2065 w2091] -> w2045
            frame "Spectrum", Default {
              n195 = local read "Suppl_3D"() -> (w2078:dbl[][][])
              n196 = local read "Detector"() -> (w2074:string)
              n197 = local read "SamplePrep"() -> (w2064:string)
              n198 = local read "Grating"() -> (w2073:string)
              n199 = local read "Marker"() -> (w2075:i8[])
              n200 = local read "SynthTemp"() -> (w2070:dbl)
              n201 = local read "SynthPolymPerc"() -> (w2067:dbl)
              n202 = local read "SynthDilution"() -> (w2069:dbl)
              n203 = local read "SynthName"() -> (w2071:string)
              n204 = local read "SampleOf"() -> (w2072:string)
              n205 = local read "SynthPolym"() -> (w2068:string)
              n206 = local read "SynthSolv"() -> (w2066:string)
              n207 = local read "FSM"() -> (w2076:dbl[])
              n208 = local read "Att"() -> (w2077:dbl[])
              n209 = local read "Main 3D Data to write"() -> (w2079:dbl[][][])
              n210 = Bundle("Date"=w2089, "Comment"=w2088, "T_K"=w2087, "ESource"=w2086, "EWL_nm"=w2085, "EPow_uW"=w2084, "Time_ms"=w2083, "WL_nm"=w2082, "Suppl_3D"=w2078, "L2Exc_deg"=w2081, "L2Det_deg"=w2080, "Att"=w2077, "FSM"=w2076, "Marker"=w2075, "Detector"=w2074, "Grating"=w2073, "SamplePrep"=w2064, "SampleOf"=w2072, "SynthName"=w2071, "SynthTemp"=w2070, "SynthDilution"=w2069, "SynthPolym"=w2068, "SynthPolymPerc"=w2067, "SynthSolv"=w2066) -> (w2065:T19)  [unwired: 1 in]
            }
            frame "Image" {
              n211 = local read "Suppl_3D"() -> (w2104:dbl[][][])
              n212 = local read "Detector"() -> (w2100:string)
              n213 = local read "Grating"() -> (w2099:string)
              n214 = local read "Marker"() -> (w2101:i8[])
              n215 = local read "SynthTemp"() -> (w2096:dbl)
              n216 = local read "SynthPolymPerc"() -> (w2093:dbl)
              n217 = local read "SynthDilution"() -> (w2095:dbl)
              n218 = local read "SynthName"() -> (w2097:string)
              n219 = local read "SampleOf"() -> (w2098:string)
              n220 = local read "SynthPolym"() -> (w2094:string)
              n221 = local read "SynthSolv"() -> (w2092:string)
              n222 = local read "Main 3D Data to write"() -> (w2105:dbl[][][])
              n223 = local read "FSM"() -> (w2102:dbl[])
              n224 = local read "Att"() -> (w2103:dbl[])
              n225 = local read "SamplePrep"() -> (w2090:string)
              n226 = Bundle("Date"=w2115, "Comment"=w2114, "T_K"=w2113, "ESource"=w2112, "EWL_nm"=w2111, "EPow_uW"=w2110, "Time_ms"=w2109, "WL_nm"=w2108, "Suppl_3D"=w2104, "L2Exc_deg"=w2107, "L2Det_deg"=w2106, "Att"=w2103, "FSM"=w2102, "Marker"=w2101, "Detector"=w2100, "Grating"=w2099, "SamplePrep"=w2090, "SampleOf"=w2098, "SynthName"=w2097, "SynthTemp"=w2096, "SynthDilution"=w2095, "SynthPolym"=w2094, "SynthPolymPerc"=w2093, "SynthSolv"=w2092) -> (w2091:T19)  [unwired: 1 in]
            }
          }
          n227 = xnode "Write Dataset with Attributes"("Dataset Path"=w2052, "error in (no error)"=w2051, "operation (open or create)"=w2050, "HDF5 Path or Ref"=w2049, "Attribute Value(s)"=w2045, "Data"=w2047) -> ("error out"=w2048:errorcluster)  [unwired: 2 in, 2 out]
        }
        frame "Spectrum" {
          n228 = local read "Acq Mode"() -> (w2456:T2)
          n229 = case shown="\"Image\"" w2456 {
            tunnel: w2472 -> [w2503 w2874 w3245 w3616 w3987]
            tunnel: w2471 -> [w2487 w2858 w3229 w3600 w3970]
            tunnel: w2470 -> [w2502 w2873 w3244 w3615 w3986]
            tunnel: w2469 -> [w2501 w2872 w3243 w3614 w3985]
            tunnel: w2468 -> [w2500 w2871 w3242 w3613 w3984]
            tunnel: w2467 -> [w2499 w2870 w3241 w3612 w3983]
            tunnel: w2466 -> [w2498 w2869 w3240 w3611 w3982]
            tunnel: w2465 -> [w2497 w2868 w3239 w3610 w3981]
            tunnel: w2464 -> [w2496 w2867 w3238 w3609 w3980]
            tunnel: w2463 -> [w2495 w2866 w3237 w3608 w3979]
            tunnel: w2462 -> [w2494 w2865 w3236 w3607 w3978]
            tunnel: w2461 -> [w2493 w2864 w3235 w3606 w3977]
            tunnel: w2460 -> [w2492 w2863 w3234 w3605 w3976]
            tunnel: w2459 -> [w2491 w2862 w3233 w3604 w3975]
            tunnel: w2458 -> [w2490 w2861 w3232 w3603 w3974]
            tunnel: [w2489 w2860 w3231 w3602 w3973] -> w2457
            frame "Spectrum", Default {
              n230 = local read "Detector"() -> (w2483:string)
              n231 = local read "Grating"() -> (w2482:string)
              n232 = local read "Marker"() -> (w2484:i8[])
              n233 = local read "SynthTemp"() -> (w2479:dbl)
              n234 = local read "SynthPolymPerc"() -> (w2476:dbl)
              n235 = local read "SynthDilution"() -> (w2478:dbl)
              n236 = local read "SynthName"() -> (w2480:string)
              n237 = local read "SampleOf"() -> (w2481:string)
              n238 = local read "SynthPolym"() -> (w2477:string)
              n239 = local read "SynthSolv"() -> (w2475:string)
              n240 = local read "FSM"() -> (w2485:dbl[])
              n241 = local read "Att"() -> (w2486:dbl[])
              n242 = local read "Data_CCD_px"() -> (w2488:dbl[][])
              n243 = local read "SamplePrep"() -> (w2473:string)
              n244 = Bundle("Date"=w2503, "Comment"=w2487, "T_K"=w2502, "ESource"=w2501, "EWL_nm"=w2500, "EPow_uW"=w2499, "Time_ms"=w2498, "WL_nm"=w2497, "Suppl"=w2496, "L2Exc_deg"=w2495, "L2Det_deg"=w2494, "Att"=w2486, "FSM"=w2485, "Marker"=w2484, "Detector"=w2483, "Grating"=w2482, "SamplePrep"=w2473, "SampleOf"=w2481, "SynthName"=w2480, "SynthTemp"=w2479, "SynthDilution"=w2478, "SynthPolym"=w2477, "SynthPolymPerc"=w2476, "SynthSolv"=w2475) -> (w2474:T15)  [unwired: 1 in]
              n245 = xnode "Write Dataset with Attributes"("Dataset Path"=w2493, "error in (no error)"=w2492, "operation (open or create)"=w2491, "HDF5 Path or Ref"=w2490, "Attribute Value(s)"=w2474, "Data"=w2488) -> ("error out"=w2489:errorcluster)  [unwired: 2 in, 2 out]
            }
            frame "APD 1" {
              n246 = local read "Detector"() -> (w2854:string)
              n247 = local read "Grating"() -> (w2853:string)
              n248 = local read "Marker"() -> (w2855:i8[])
              n249 = local read "FSM"() -> (w2856:dbl[])
              n250 = local read "Att"() -> (w2857:dbl[])
              n251 = local read "SynthTemp"() -> (w2850:dbl)
              n252 = local read "SynthPolymPerc"() -> (w2847:dbl)
              n253 = local read "SynthDilution"() -> (w2849:dbl)
              n254 = local read "SynthName"() -> (w2851:string)
              n255 = local read "SampleOf"() -> (w2852:string)
              n256 = local read "SynthPolym"() -> (w2848:string)
              n257 = local read "SynthSolv"() -> (w2846:string)
              n258 = local read "Data_CCD_px"() -> (w2859:dbl[][])
              n259 = local read "SamplePrep"() -> (w2844:string)
              n260 = Bundle("Date"=w2874, "Comment"=w2858, "T_K"=w2873, "ESource"=w2872, "EWL_nm"=w2871, "EPow_uW"=w2870, "Time_ms"=w2869, "WL_nm"=w2868, "Suppl"=w2867, "L2Exc_deg"=w2866, "L2Det_deg"=w2865, "Att"=w2857, "FSM"=w2856, "Marker"=w2855, "Detector"=w2854, "Grating"=w2853, "SamplePrep"=w2844, "SampleOf"=w2852, "SynthName"=w2851, "SynthTemp"=w2850, "SynthDilution"=w2849, "SynthPolym"=w2848, "SynthPolymPerc"=w2847, "SynthSolv"=w2846) -> (w2845:T15)  [unwired: 1 in]
              n261 = xnode "Write Dataset with Attributes"("Dataset Path"=w2864, "error in (no error)"=w2863, "operation (open or create)"=w2862, "HDF5 Path or Ref"=w2861, "Attribute Value(s)"=w2845, "Data"=w2859) -> ("error out"=w2860:errorcluster)  [unwired: 2 in, 2 out]
            }
            frame "APD 2" {
              n262 = local read "Detector"() -> (w3225:string)
              n263 = local read "Grating"() -> (w3224:string)
              n264 = local read "Marker"() -> (w3226:i8[])
              n265 = local read "SynthTemp"() -> (w3221:dbl)
              n266 = local read "SynthPolymPerc"() -> (w3218:dbl)
              n267 = local read "SynthDilution"() -> (w3220:dbl)
              n268 = local read "SynthName"() -> (w3222:string)
              n269 = local read "SampleOf"() -> (w3223:string)
              n270 = local read "SynthPolym"() -> (w3219:string)
              n271 = local read "SynthSolv"() -> (w3217:string)
              n272 = local read "FSM"() -> (w3227:dbl[])
              n273 = local read "Att"() -> (w3228:dbl[])
              n274 = local read "SamplePrep"() -> (w3215:string)
              n275 = local read "Data_CCD_px"() -> (w3230:dbl[][])
              n276 = Bundle("Date"=w3245, "Comment"=w3229, "T_K"=w3244, "ESource"=w3243, "EWL_nm"=w3242, "EPow_uW"=w3241, "Time_ms"=w3240, "WL_nm"=w3239, "Suppl"=w3238, "L2Exc_deg"=w3237, "L2Det_deg"=w3236, "Att"=w3228, "FSM"=w3227, "Marker"=w3226, "Detector"=w3225, "Grating"=w3224, "SamplePrep"=w3215, "SampleOf"=w3223, "SynthName"=w3222, "SynthTemp"=w3221, "SynthDilution"=w3220, "SynthPolym"=w3219, "SynthPolymPerc"=w3218, "SynthSolv"=w3217) -> (w3216:T15)  [unwired: 1 in]
              n277 = xnode "Write Dataset with Attributes"("Dataset Path"=w3235, "error in (no error)"=w3234, "operation (open or create)"=w3233, "HDF5 Path or Ref"=w3232, "Attribute Value(s)"=w3216, "Data"=w3230) -> ("error out"=w3231:errorcluster)  [unwired: 2 in, 2 out]
            }
            frame "APD 1+2" {
              n278 = local read "Detector"() -> (w3596:string)
              n279 = local read "Grating"() -> (w3595:string)
              n280 = local read "Marker"() -> (w3597:i8[])
              n281 = local read "FSM"() -> (w3598:dbl[])
              n282 = local read "Att"() -> (w3599:dbl[])
              n283 = local read "SynthTemp"() -> (w3592:dbl)
              n284 = local read "SynthPolymPerc"() -> (w3589:dbl)
              n285 = local read "SynthDilution"() -> (w3591:dbl)
              n286 = local read "SynthName"() -> (w3593:string)
              n287 = local read "SampleOf"() -> (w3594:string)
              n288 = local read "SynthPolym"() -> (w3590:string)
              n289 = local read "SynthSolv"() -> (w3588:string)
              n290 = local read "Data_CCD_px"() -> (w3601:dbl[][])
              n291 = local read "SamplePrep"() -> (w3586:string)
              n292 = Bundle("Date"=w3616, "Comment"=w3600, "T_K"=w3615, "ESource"=w3614, "EWL_nm"=w3613, "EPow_uW"=w3612, "Time_ms"=w3611, "WL_nm"=w3610, "Suppl"=w3609, "L2Exc_deg"=w3608, "L2Det_deg"=w3607, "Att"=w3599, "FSM"=w3598, "Marker"=w3597, "Detector"=w3596, "Grating"=w3595, "SamplePrep"=w3586, "SampleOf"=w3594, "SynthName"=w3593, "SynthTemp"=w3592, "SynthDilution"=w3591, "SynthPolym"=w3590, "SynthPolymPerc"=w3589, "SynthSolv"=w3588) -> (w3587:T15)  [unwired: 1 in]
              n293 = xnode "Write Dataset with Attributes"("Dataset Path"=w3606, "error in (no error)"=w3605, "operation (open or create)"=w3604, "HDF5 Path or Ref"=w3603, "Attribute Value(s)"=w3587, "Data"=w3601) -> ("error out"=w3602:errorcluster)  [unwired: 2 in, 2 out]
            }
            frame "Image" {
              n294 = local read "Detector"() -> (w3966:string)
              n295 = local read "WL_nm"() -> (w3972:sgl[])
              n296 = local read "Grating"() -> (w3965:string)
              n297 = local read "Marker"() -> (w3967:i8[])
              n298 = local read "SynthTemp"() -> (w3962:dbl)
              n299 = local read "SynthPolymPerc"() -> (w3959:dbl)
              n300 = local read "SynthDilution"() -> (w3961:dbl)
              n301 = local read "SynthName"() -> (w3963:string)
              n302 = local read "SampleOf"() -> (w3964:string)
              n303 = local read "SynthPolym"() -> (w3960:string)
              n304 = local read "Main 3D Data to write"() -> (w3971:dbl[][][])
              n305 = local read "SynthSolv"() -> (w3958:string)
              n306 = local read "FSM"() -> (w3968:dbl[])
              n307 = local read "Att"() -> (w3969:dbl[])
              n308 = local read "SamplePrep"() -> (w3957:string)
              n309 = Bundle("Date"=w3987, "Comment"=w3970, "T_K"=w3986, "ESource"=w3985, "EWL_nm"=w3984, "EPow_uW"=w3983, "Time_ms"=w3982, "WL_nm"=w3981, "Suppl"=w3980, "L2Exc_deg"=w3979, "L2Det_deg"=w3978, "WL_nm"=w3972, "Att"=w3969, "FSM"=w3968, "Marker"=w3967, "Detector"=w3966, "Grating"=w3965, "SamplePrep"=w3957, "SampleOf"=w3964, "SynthName"=w3963, "SynthTemp"=w3962, "SynthDilution"=w3961, "SynthPolym"=w3960, "SynthPolymPerc"=w3959, "SynthSolv"=w3958) -> ()  [unwired: 1 in, 1 out]
              n310 = xnode "Write Dataset with Attributes"("Dataset Path"=w3977, "error in (no error)"=w3976, "operation (open or create)"=w3975, "HDF5 Path or Ref"=w3974, "Data"=w3971) -> ("error out"=w3973:errorcluster)  [unwired: 3 in, 2 out]
            }
          }
        }
        frame "Time Trace" {
          n311 = local read "Acq Mode"() -> (w4282:T2)
          n312 = case shown="\"Spectrum\", Default" w4282 {
            tunnel: w4298 -> [w4327 w4694]
            tunnel: w4297 -> [w4326 w4693]
            tunnel: w4296 -> [w4325 w4692]
            tunnel: w4295 -> [w4324 w4691]
            tunnel: w4294 -> [w4323 w4690]
            tunnel: w4293 -> [w4322 w4689]
            tunnel: w4292 -> [w4321 w4688]
            tunnel: w4291 -> [w4320 w4687]
            tunnel: w4290 -> [w4319 w4686]
            tunnel: w4289 -> [w4318 w4685]
            tunnel: w4288 -> [w4317 w4684]
            tunnel: w4287 -> [w4316 w4683]
            tunnel: w4286 -> [w4315 w4682]
            tunnel: w4285 -> [w4314 w4681]
            tunnel: w4284 -> [w4313 w4680]
            tunnel: [w4312 w4679] -> w4283
            frame "Spectrum", Default {
              n313 = local read "Marker"() -> (w4308:i8[])
              n314 = local read "FSM"() -> (w4309:dbl[])
              n315 = local read "Att"() -> (w4310:dbl[])
              n316 = local read "SynthTemp"() -> (w4305:dbl)
              n317 = local read "SynthPolymPerc"() -> (w4302:dbl)
              n318 = local read "SynthDilution"() -> (w4304:dbl)
              n319 = local read "SynthName"() -> (w4306:string)
              n320 = local read "SampleOf"() -> (w4307:string)
              n321 = local read "SynthPolym"() -> (w4303:string)
              n322 = local read "SynthSolv"() -> (w4301:string)
              n323 = local read "SamplePrep"() -> (w4299:string)
              n324 = local read "Data_CCD_px"() -> (w4311:dbl[][])
              n325 = Bundle("Date"=w4327, "Comment"=w4326, "T_K"=w4325, "ESource"=w4324, "EWL_nm"=w4323, "EPow_uW"=w4322, "Time_ms"=w4321, "WL_nm"=w4320, "Suppl"=w4319, "L2Exc_deg"=w4318, "L2Det_deg"=w4317, "Att"=w4310, "FSM"=w4309, "Marker"=w4308, "SamplePrep"=w4299, "SampleOf"=w4307, "SynthName"=w4306, "SynthTemp"=w4305, "SynthDilution"=w4304, "SynthPolym"=w4303, "SynthPolymPerc"=w4302, "SynthSolv"=w4301) -> (w4300:T20)  [unwired: 1 in]
              n326 = xnode "Write Dataset with Attributes"("Dataset Path"=w4316, "error in (no error)"=w4315, "operation (open or create)"=w4314, "HDF5 Path or Ref"=w4313, "Attribute Value(s)"=w4300, "Data"=w4311) -> ("error out"=w4312:errorcluster)  [unwired: 2 in, 2 out]
            }
            frame "Image" {
              n327 = local read "Detector"() -> (w4674:string)
              n328 = local read "Grating"() -> (w4673:string)
              n329 = local read "Marker"() -> (w4675:i8[])
              n330 = local read "FSM"() -> (w4676:dbl[])
              n331 = local read "Att"() -> (w4677:dbl[])
              n332 = local read "SynthTemp"() -> (w4670:dbl)
              n333 = local read "SynthPolymPerc"() -> (w4667:dbl)
              n334 = local read "SynthDilution"() -> (w4669:dbl)
              n335 = local read "SynthName"() -> (w4671:string)
              n336 = local read "SampleOf"() -> (w4672:string)
              n337 = local read "SynthPolym"() -> (w4668:string)
              n338 = local read "SynthSolv"() -> (w4666:string)
              n339 = local read "Main 3D Data to write"() -> (w4678:dbl[][][])
              n340 = local read "SamplePrep"() -> (w4664:string)
              n341 = Bundle("Date"=w4694, "Comment"=w4693, "T_K"=w4692, "ESource"=w4691, "EWL_nm"=w4690, "EPow_uW"=w4689, "Time_ms"=w4688, "WL_nm"=w4687, "Suppl"=w4686, "L2Exc_deg"=w4685, "L2Det_deg"=w4684, "Att"=w4677, "FSM"=w4676, "Marker"=w4675, "Detector"=w4674, "Grating"=w4673, "SamplePrep"=w4664, "SampleOf"=w4672, "SynthName"=w4671, "SynthTemp"=w4670, "SynthDilution"=w4669, "SynthPolym"=w4668, "SynthPolymPerc"=w4667, "SynthSolv"=w4666) -> (w4665:T15)  [unwired: 1 in]
              n342 = xnode "Write Dataset with Attributes"("Dataset Path"=w4683, "error in (no error)"=w4682, "operation (open or create)"=w4681, "HDF5 Path or Ref"=w4680, "Attribute Value(s)"=w4665, "Data"=w4678) -> ("error out"=w4679:errorcluster)  [unwired: 2 in, 2 out]
            }
          }
        }
        frame "XY Intensity Map" {
          n343 = local read "Suppl_2D"() -> (w5049:dbl[][])
          n344 = local read "Detector"() -> (w5045:string)
          n345 = local read "Grating"() -> (w5044:string)
          n346 = local read "Marker"() -> (w5046:i8[])
          n347 = local read "SynthTemp"() -> (w5041:dbl)
          n348 = local read "SynthPolymPerc"() -> (w5038:dbl)
          n349 = local read "SynthDilution"() -> (w5040:dbl)
          n350 = local read "SynthName"() -> (w5042:string)
          n351 = local read "SampleOf"() -> (w5043:string)
          n352 = local read "SynthPolym"() -> (w5039:string)
          n353 = local read "SynthSolv"() -> (w5037:string)
          n354 = local read "SamplePrep"() -> (w5036:string)
          n355 = local read "FSM"() -> (w5047:dbl[])
          n356 = local read "Att"() -> (w5048:dbl[])
          n357 = Bundle("Date"=w5066, "Comment"=w5065, "T_K"=w5064, "ESource"=w5063, "EWL_nm"=w5062, "EPow_uW"=w5061, "Time_ms"=w5060, "WL_nm"=w5059, "Suppl"=w5058, "L2Exc_deg"=w5057, "L2Det_deg"=w5056, "Suppl_2D"=w5049, "Att"=w5048, "FSM"=w5047, "Marker"=w5046, "Detector"=w5045, "Grating"=w5044, "SamplePrep"=w5036, "SampleOf"=w5043, "SynthName"=w5042, "SynthTemp"=w5041, "SynthDilution"=w5040, "SynthPolym"=w5039, "SynthPolymPerc"=w5038, "SynthSolv"=w5037) -> (w5035:T17)  [unwired: 1 in]
          n358 = local read "Data_CCD_px"() -> (w5050:dbl[][])
          n359 = xnode "Write Dataset with Attributes"("Dataset Path"=w5055, "error in (no error)"=w5054, "operation (open or create)"=w5053, "HDF5 Path or Ref"=w5052, "Attribute Value(s)"=w5035, "Data"=w5050) -> ("error out"=w5051:errorcluster)  [unwired: 2 in, 2 out]
        }
      }
      n360 = Concatenate Strings("Data written to file ", w93, " as ", w91) -> (w89:string)
      n361 = call "Write2LogFile.vi"("Add to log file"=w89, "Log file before"=w90, "Checkbox"=FALSE) -> ("Log file after"=w88:string)
      n362 = local write "Log File Out"(w88) -> ()
      n363 = disable-structure shown="Disabled" {
        frame Disabled {
          n364 = local read "SamplePrepdate"() -> ()  [unwired: 1 out]
          n365 = local read "SynthTemp"() -> ()  [unwired: 1 out]
          n366 = local read "SynthPolymPerc"() -> ()  [unwired: 1 out]
          n367 = local read "SynthDilution"() -> ()  [unwired: 1 out]
          n368 = local read "SynthName"() -> ()  [unwired: 1 out]
          n369 = local read "SampleOf"() -> ()  [unwired: 1 out]
          n370 = local read "SynthPolym"() -> ()  [unwired: 1 out]
          n371 = local read "SynthSolv"() -> ()  [unwired: 1 out]
        }
        frame Enabled {
        }
      }
      n372 = call <vilib>:"H5Fclose.vi"("error in (no error)"=w124, "Close All Open Objects (T)"=TRUE, "HDF5 Ref"=w101) -> ("error out"=w99:errorcluster)  [unwired: 6 in]
      n373 = call <vilib>:"Recover Error Stack.vi"("error in (no error)"=w99) -> ()  [unwired: 5 in, 4 out]
      "File path" <- w82
    }
  }
  n374 = local read "Data_PLInt_cts"() -> (w6:i32[])
  n375 = local read "WL_nm"() -> (w5:sgl[])
  n376 = Bundle("WL_nm"=w5, "Data_PLInt_cts"=w6) -> ()  [unwired: 1 in, 1 out]
